vi "Treshold_Finder.vi"() -> ()   [LabVIEW 2012]
panel:
  out "8bit integer":i8
  out "Maximo - Minimo 3":dbl[](array[numeric])
  out "element":dbl
  out "Maximo - Minimo 2":dbl[](array[numeric])
  in  "Values":dbl[](array[numeric])
  in  "Maximo - Minimo":u16[](array[numeric])
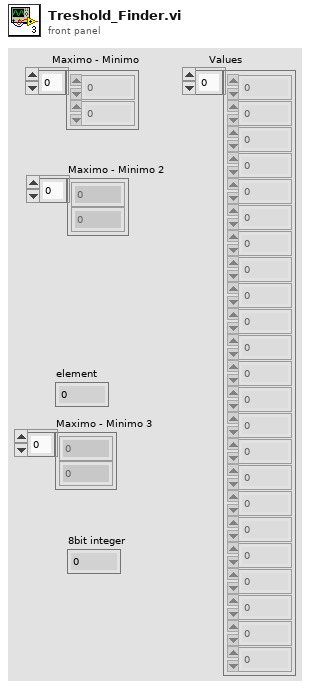
[diagram p1: front panel]
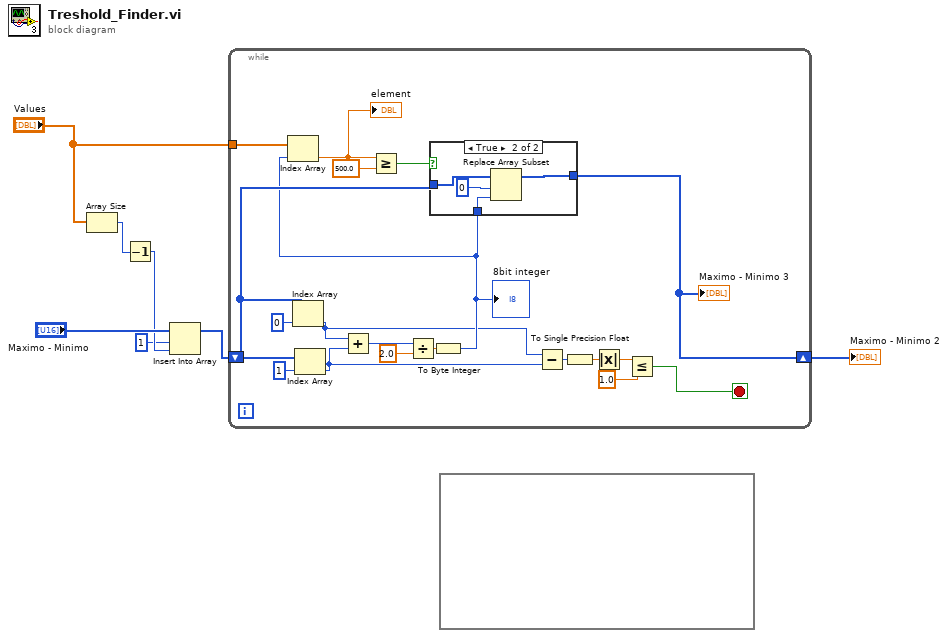
[diagram p0: block diagram]
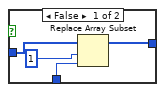
[diagram p2: hidden frame]
diagram:
  n1 = Array Size(array="Values") -> (size(s)=w7:i32)
  n2 = Decrement(x=w7) -> (x-1=w5:i32)
  n3 = Insert Into Array(array="Maximo - Minimo", index=1, new element=w5) -> (w3:u16[])
  n4 = while {
    shift-right: [w17] -> w2
    shift-left: w3 -> [w18]
    tunnel: "Values" -> [w22]
    stop <- w8 stop-if-true
    n5 = Index Array(array=w18, index=0) -> (element=w14:u16)
    n6 = Index Array(array=w18, index=1) -> (element=w13:u16)
    n7 = Add(x=w14, y=w13) -> (x+y=w24:u16)
    n8 = Divide(x=w24, y=2.0) -> (x/y=w16:dbl)
    n9 = To Byte Integer(number=w16) -> (8bit integer=w15:i8)
    "8bit integer" <- w15
    n10 = Index Array(array=w22, index=w15) -> (element=w21:dbl)
    "element" <- w21
    n11 = Greater Or Equal?(x=w21, y=500.0) -> (x >= y?=w19:bool)
    n12 = case shown="True" w19 {
      tunnel: w18 -> [w28 w33]
      tunnel: [w27 w34] -> w17
      tunnel: w15 -> [w30 w31]
      frame False {
        n13 = Replace Array Subset(array=w28, new element=w30, index=1) -> (w27:u16[])
      }
      frame True {
        n14 = Replace Array Subset(array=w33, new element=w31, index=0) -> (w34:u16[])
      }
    }
    "Maximo - Minimo 3" <- w17
    n15 = Subtract(x=w14, y=w13) -> (x-y=w12:u16)
    n16 = To Single Precision Float(number=w12) -> (single precision float=w11:sgl)
    n17 = Absolute Value(x=w11) -> (abs(x)=w10:sgl)
    n18 = Less Or Equal?(x=w10, y=sgl 1.0) -> (x <= y?=w8:bool)
  }
  "Maximo - Minimo 2" <- w2
  n19 = formula code=""() -> ()
